vi "generate_children.vi"(8 "Error In":errorcluster, 11 "GenAlg_data":T1) -> (0 "Error Out":errorcluster, 3 "GenAlg_data-out":T1)   [LabVIEW 2016]
uses:
  TypeDefs/GenAlg_data.ctl
  TypeDefs/basic_config.ctl
  TypeDefs/element.ctl
  TypeDefs/geration_data.ctl
  TypeDefs/selection_data.ctl
  TypeDefs/SimulatedAnnealing_data.ctl
  TypeDefs/multi_eval_data.ctl
  TypeDefs/termination_data.ctl
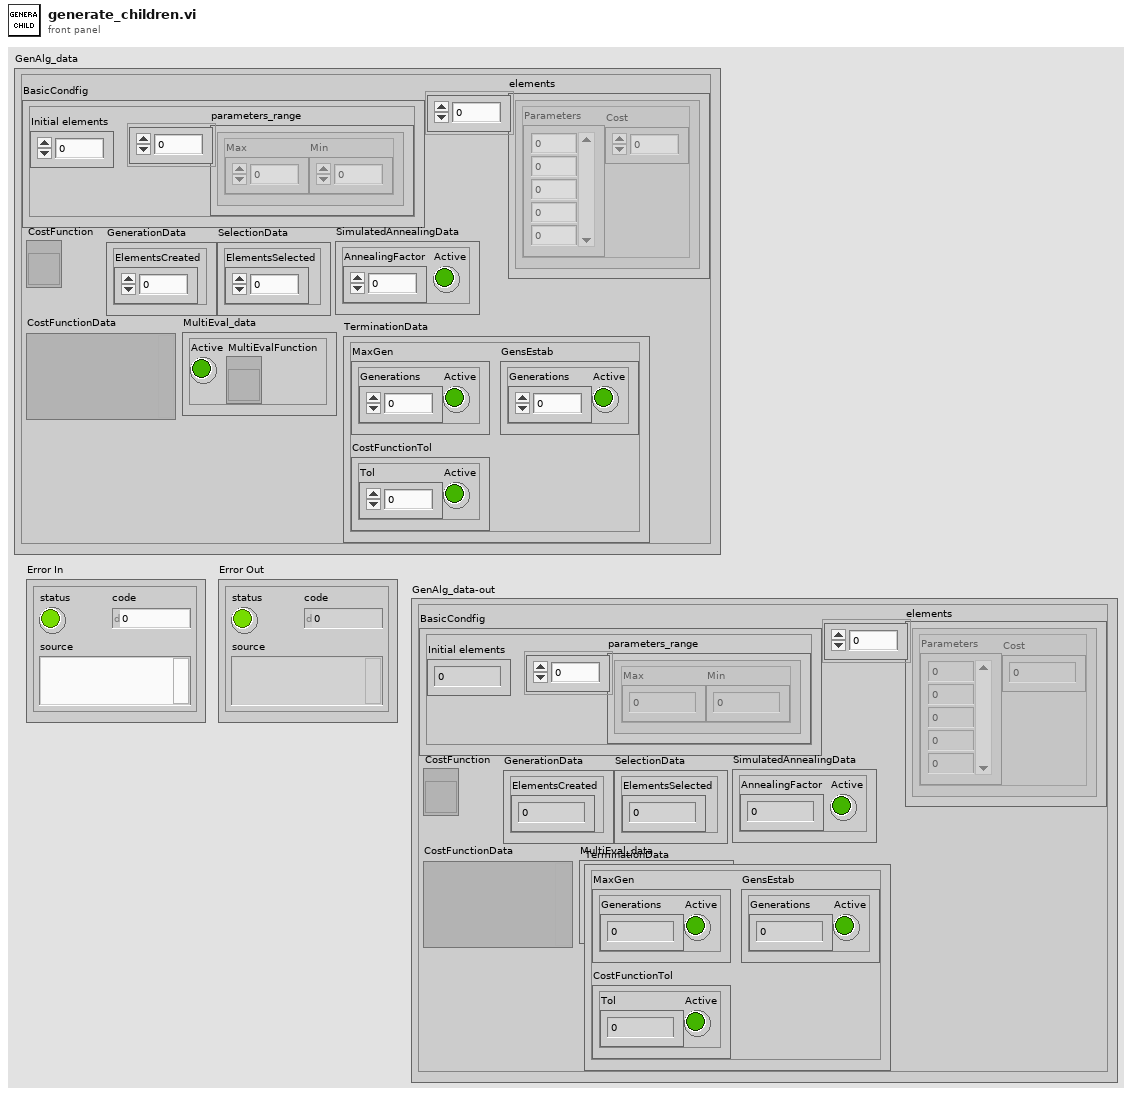
[diagram p1: front panel]
types:
  T1 = typedef "GenAlg_data.ctl" = cluster{"BasicCondfig":T2, "elements":T3[], "CostFunction":refnum<vi>, "GenerationData":T4, "SelectionData":T5, "SimulatedAnnealingData":T6, "CostFunctionData":variant, "MultiEval_data":T7, "TerminationData":T8}
  T2 = typedef "basic_config.ctl" = cluster{"parameters_range":cluster{"Max":dbl, "Min":dbl}[], "Initial elements":i32}
  T3 = typedef "element.ctl" = cluster{"Parameters":dbl[], "Cost":dbl}
  T4 = typedef "geration_data.ctl" = cluster{"ElementsCreated":i32}
  T5 = typedef "selection_data.ctl" = cluster{"ElementsSelected":i32}
  T6 = typedef "SimulatedAnnealing_data.ctl" = cluster{"AnnealingFactor":dbl, "Active":bool}
  T7 = typedef "multi_eval_data.ctl" = cluster{"Active":bool, "MultiEvalFunction":refnum<vi>}
  T8 = typedef "termination_data.ctl" = cluster{"MaxGen":cluster{"Generations":i32, "Active":bool}, "CostFunctionTol":cluster{"Tol":dbl, "Active":bool}, "GensEstab":cluster{"Generations":i32, "Active":bool}}
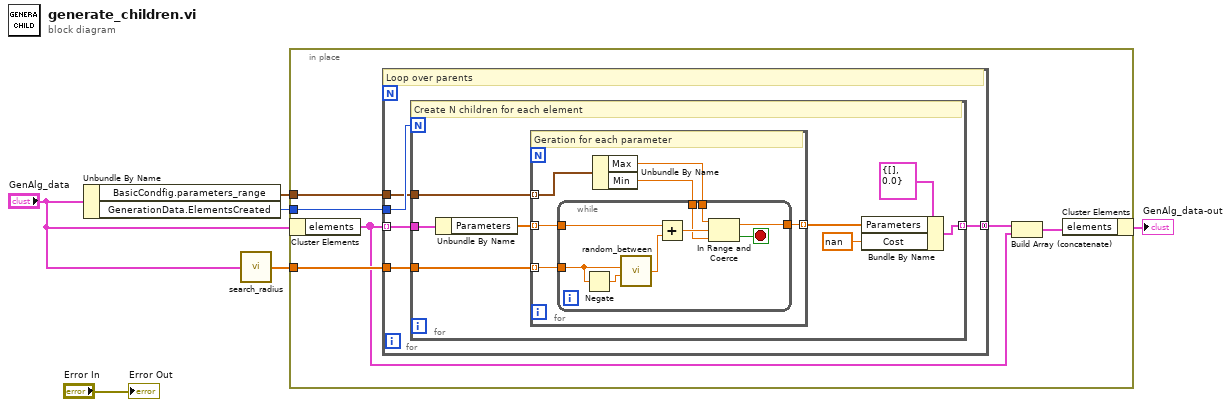
[diagram p0: block diagram]
diagram:
  n1 = Unbundle By Name("GenAlg_data") -> ("BasicCondfig.parameters_range"=w4:cluster{"Max":dbl, "Min":dbl}[], "GenerationData.ElementsCreated"=w6:i32)
  n2 = call "search_radius.vi"("GenAlg_data"="GenAlg_data") -> ("Radius"=w5:dbl[])
  n3 = in-place {
    in-place-border: w6 -> [w12]
    in-place-border: w5 -> [w11]
    in-place-border: w4 -> [w10]
    n4 = in-place-cluster #1("GenAlg_data") -> ("elements"=w8:T3[])
    n5 = for {
      tunnel: w8 -> [w15] mode=indexing
      tunnel: w12 -> [w17]
      tunnel: w11 -> [w16]
      tunnel: w10 -> [w14]
      tunnel: [w13] -> w9 mode=concatenating
      # "Loop over parents"
      n6 = for {
        N: w17 -> [_]
        tunnel: w15 -> [w24]
        tunnel: w16 -> [w25]
        tunnel: w14 -> [w22]
        tunnel: [w19] -> w13 mode=indexing
        # "Create N children for each element"
        n7 = Unbundle By Name(w24) -> ("Parameters"=w23:dbl[])
        n8 = for {
          tunnel: w25 -> [w31] mode=indexing
          tunnel: w23 -> [w30] mode=indexing
          tunnel: w22 -> [w29] mode=indexing
          tunnel: [w26] -> w20 mode=indexing
          # "Geration for each parameter"
          n9 = Unbundle By Name(w29) -> ("Max"=w27:dbl, "Min"=w28:dbl)
          n10 = while {
            tunnel: w31 -> [w39]
            tunnel: w30 -> [w37]
            tunnel: w28 -> [w35]
            tunnel: w27 -> [w34]
            tunnel: [w32] -> w26
            stop <- w33 stop-if-true
            n11 = Negate(x=w39) -> (-x=w40:dbl)
            n12 = call "random_between.vi"("b"=w40, "a"=w39) -> ("Random"=w38:dbl)  [unwired: 4 in]
            n13 = Add(x=w37, y=w38) -> (x+y=w36:dbl)
            n14 = In Range and Coerce(upper limit=w34, x=w36, lower limit=w35) -> (coerced(x)=w32:dbl, In Range?=w33:bool)
          }
        }
        n15 = Bundle By Name(cluster=T3 {"Parameters"=[], "Cost"=0.0} ("element"), "Parameters"=w20, "Cost"=nan) -> (w19:T3)
      }
    }
    n16 = Build Array (concatenate)(w9, w8) -> (w7:T3[])
    n17 = in-place-cluster #1("elements"=w7) -> (→"GenAlg_data-out":T1)
  }
  "Error Out" <- "Error In"
